vi "SubVI_SVM_Linear Kernel.vi"(11 "X":dbl[][](array[numeric])) -> (3 "K":T1)   [LabVIEW 2020]
uses:
  <vilib>/Analysis/Matrix/Datatypes/RealMatrix.ctl
  <vilib>/Analysis/baseanly.llb/Real A x B.vi
  <vilib>/Analysis/NI_AALBase.lvlib
  <vilib>/Analysis/Matrix/NI_Matrix.lvlib
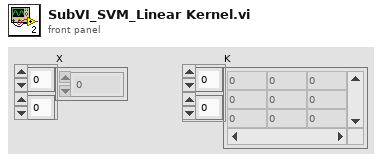
[diagram p1: front panel]
types:
  T1 = typedef "NI_Matrix.lvlib/RealMatrix.ctl" = dbl[][]
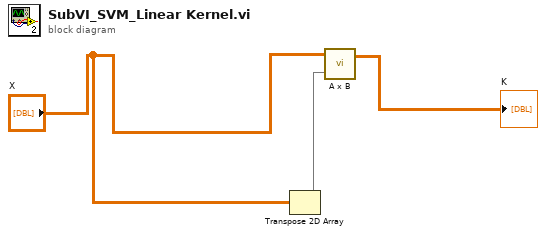
[diagram p0: block diagram]
diagram:
  n1 = Transpose 2D Array(2D array="X") -> (transposed array=w2:dbl[][])
  n2 = call-poly <vilib>:"A x B.vi"("B"=w2, "A"="X") -> ("A x B"=→"K":T1)  [unwired: 1 out]
